vi "[PC]MainGUI_Engineering.vi"() -> ()   [LabVIEW 2018]
doc: "Das soll ein Frontpanel sein, welches einem die aktuellsten internen Parameter angibt wie zB. einen Temperaturverlaufsgraph."
uses:
  TypeDef/ControllerState.ctl
  RT/[GlobVar]SensorState.vi
panel:
  out "Umgebungsdruck":dbl(slide) scale=0.0..1.5 scale format="%#_g bar"
  out "Luftfeuchtigkeit":dbl(slide) scale=0.0..100.0 scale format="%#_g %"
  out "Raum Temp":dbl(slide) scale=0.0..40.0 scale format="%#_g °C"
  out "Temperatur Sieb (PT100)":dbl(slide) scale=0.0..100.0
  out "Volumen-Verlauf":dbl(graph)
  out "State Current":T1
  out "Heizer":bool
  out "Ventil":bool
  out "Sieb-Kaffe vorhanden":bool
  out "Tank":u8(slide) scale=0.0..1.0
  in  "Emg Stop":bool caption="STOP"
  out "Temperatur-Verlauf":T2(graph)
  out "Druck-Verlauf":dbl(graph)
  in  "stop":bool
  out "Kaffeetasse vorhanden":bool
  out "Wartungsklappe zu":bool
  out "Tür Hinten zu":bool
  out "Volume (ml)":dbl(knob) scale=0.0..250.0
  out "Volumen erreicht":bool
  out "Temperatur erreicht":bool
  out "Pumpe":bool
  out "Druck (psi)":dbl(slide) scale=0.0..30.0
  out "Temperatur Siedebad":dbl(slide) scale=0.0..100.0
  # "Digital Switches"
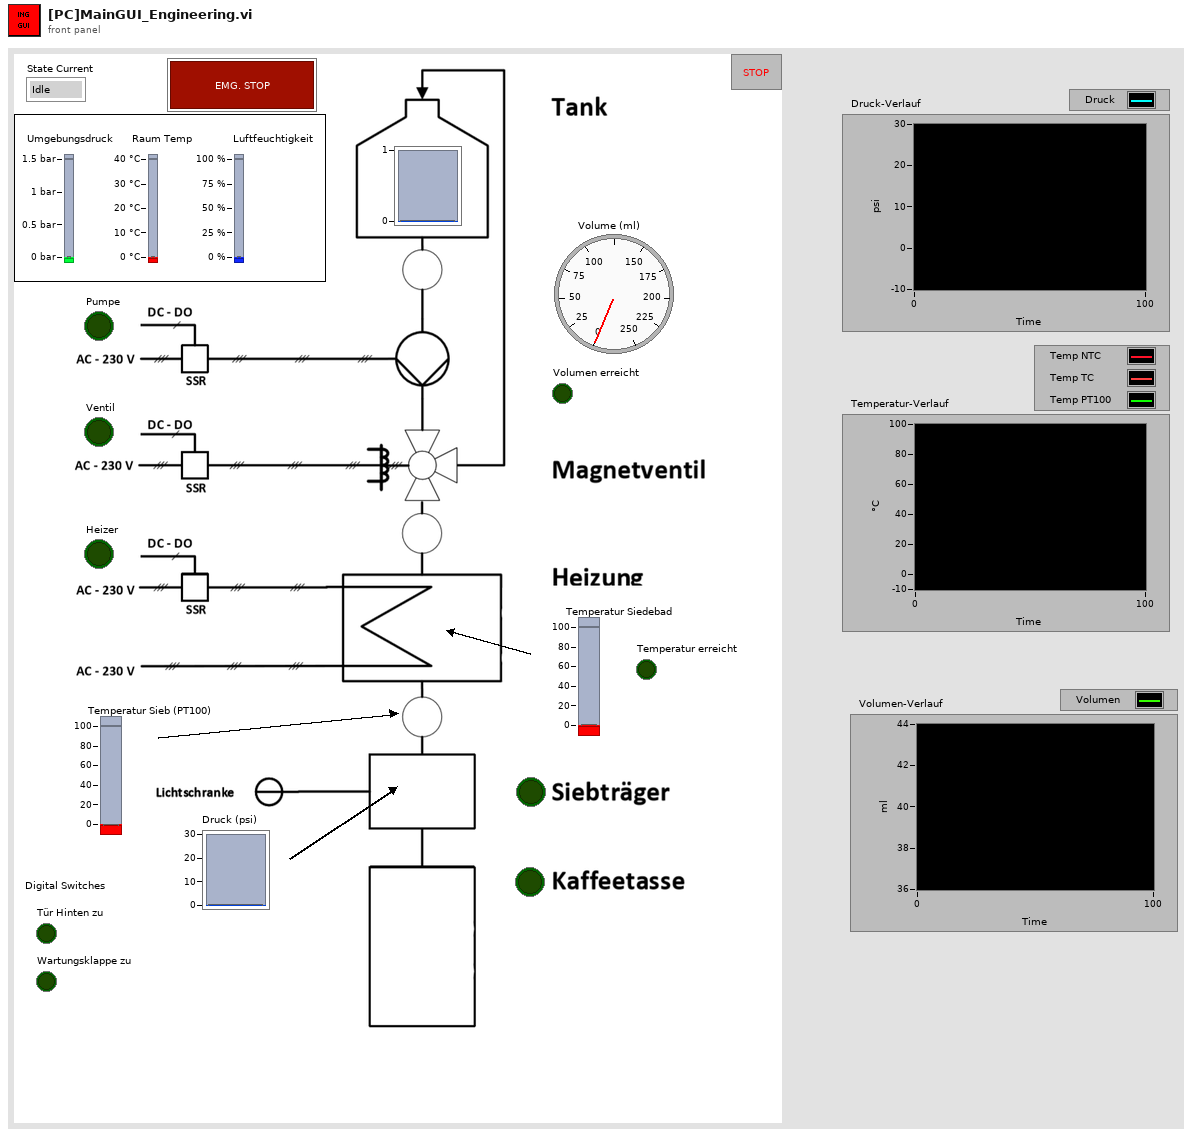
[diagram p1: front panel]
types:
  T1 = typedef "ControllerState.ctl" = enum16{"Idle", "Vorheizen", "Brühen", "Emergency-Stop"}
  T2 = cluster{"Temp_NTC":dbl, "Temp_TC":dbl, "Temp_PT100":dbl}
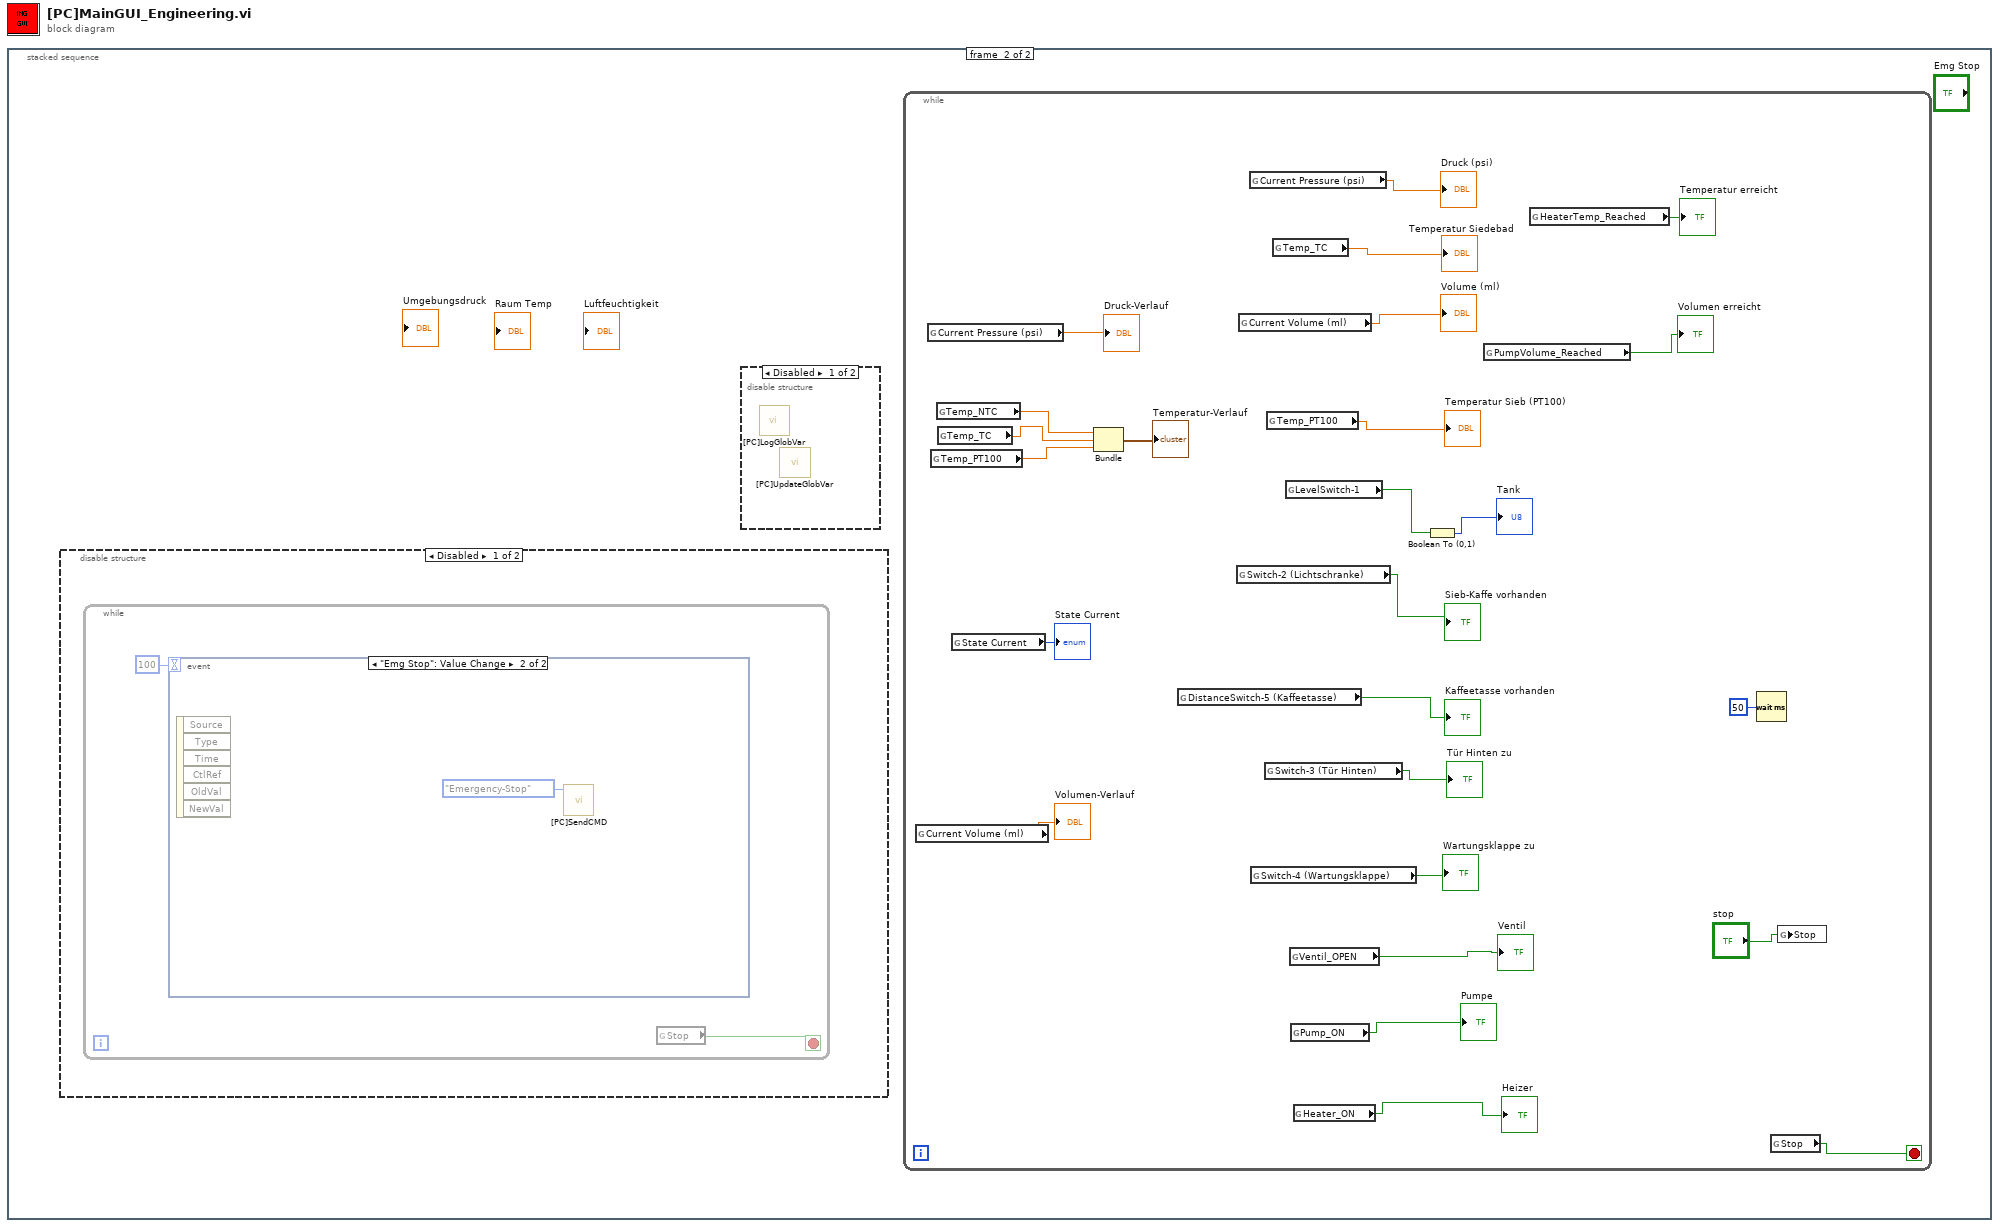
[diagram p0: block diagram]
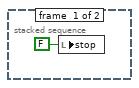
[diagram p2: hidden frame]
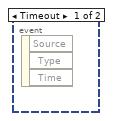
[diagram p3: hidden frame]
diagram:
  n1 = stacked-sequence {
    frame #0 {
      n2 = local write "stop"(FALSE ("stop")) -> ()
    }
    frame #1 {
      n3 = disable-structure shown="Disabled" {
        frame Disabled {
          n4 = while {
            stop <- w2 stop-if-true
            n5 = event shown="[1] \"Emg Stop\": Value Change" {
              selector: _ -> [_ _]
              dyn-events: _ -> [_ _]
              timeout: 100 -> [_ _]
              event Timeout {
                n6 = event-data() -> ()  [unwired: 1 in, 3 out]
              }
              event "Emg Stop": Value Change {
                n7 = event-data() -> ()  [unwired: 1 in, 6 out]
                n8 = call "[PC]SendCMD.vi"("State Rqst"=ControllerState."Emergency-Stop") -> ()  [unwired: 11 in]
              }
            }
            n9 = global read "[GlobVar]SensorState.vi" "Stop"() -> (w2:bool)
          }
        }
        frame Enabled {
        }
      }
      n10 = disable-structure shown="Disabled" {
        frame Disabled {
          n11 = call "[PC]LogGlobVar.vi"() -> ()  [unwired: 12 in]
          n12 = call "[PC]UpdateGlobVar.vi"() -> ()  [unwired: 12 in]
        }
        frame Enabled {
        }
      }
      n13 = while {
        stop <- w29 stop-if-true
        n14 = global read "[GlobVar]SensorState.vi" "Current Volume (ml)"() -> (→"Volumen-Verlauf":dbl)
        n15 = global read "[GlobVar]SensorState.vi" "Current Pressure (psi)"() -> (→"Druck-Verlauf":dbl)
        n16 = global read "[GlobVar]SensorState.vi" "Temp_PT100"() -> (w8:dbl)
        n17 = global read "[GlobVar]SensorState.vi" "Temp_NTC"() -> (w6:dbl)
        n18 = global read "[GlobVar]SensorState.vi" "Temp_TC"() -> (w7:dbl)
        n19 = global read "[GlobVar]SensorState.vi" "State Current"() -> (→"State Current":T1)
        n20 = Bundle("Temp_NTC"=w6, "Temp_TC"=w7, "Temp_PT100"=w8) -> (→"Temperatur-Verlauf":T2)  [unwired: 1 in]
        n21 = global read "[GlobVar]SensorState.vi" "DistanceSwitch-5 (Kaffeetasse)"() -> (→"Kaffeetasse vorhanden":bool)
        n22 = global read "[GlobVar]SensorState.vi" "Switch-2 (Lichtschranke)"() -> (→"Sieb-Kaffe vorhanden":bool)
        n23 = global read "[GlobVar]SensorState.vi" "Current Volume (ml)"() -> (→"Volume (ml)":dbl)
        n24 = global read "[GlobVar]SensorState.vi" "Current Pressure (psi)"() -> (→"Druck (psi)":dbl)
        n25 = global read "[GlobVar]SensorState.vi" "Switch-4 (Wartungsklappe)"() -> (→"Wartungsklappe zu":bool)
        n26 = global read "[GlobVar]SensorState.vi" "Switch-3 (Tür Hinten)"() -> (→"Tür Hinten zu":bool)
        n27 = global read "[GlobVar]SensorState.vi" "Temp_PT100"() -> (→"Temperatur Sieb (PT100)":dbl)
        n28 = global read "[GlobVar]SensorState.vi" "Temp_TC"() -> (→"Temperatur Siedebad":dbl)
        n29 = global read "[GlobVar]SensorState.vi" "LevelSwitch-1"() -> (w17:bool)
        n30 = global read "[GlobVar]SensorState.vi" "Ventil_OPEN"() -> (→"Ventil":bool)
        n31 = global read "[GlobVar]SensorState.vi" "Pump_ON"() -> (→"Pumpe":bool)
        n32 = global read "[GlobVar]SensorState.vi" "Heater_ON"() -> (→"Heizer":bool)
        n33 = Boolean To (0,1)(Boolean=w17) -> (0, 1=→"Tank":i16)
        n34 = global read "[GlobVar]SensorState.vi" "PumpVolume_Reached"() -> (→"Volumen erreicht":bool)
        n35 = global read "[GlobVar]SensorState.vi" "HeaterTemp_Reached"() -> (→"Temperatur erreicht":bool)
        n36 = Wait (ms)(milliseconds to wait=u32 50) -> ()  [unwired: 1 out]
        n37 = global read "[GlobVar]SensorState.vi" "Stop"() -> (w29:bool)
        n38 = global write "[GlobVar]SensorState.vi" "Stop"("stop") -> ()
      }
    }
  }
